vi "axis_angle_to_rotation.vi"(8 "Angle":dbl format="%.5f", 11 "Axis":dbl[](array[numeric])) -> (2 "Rotation":T1=[[1.0, 0.0, 0.0], [0.0, 1.0, 0.0], [0.0, 0.0, 1.0]] format="%#_4g")   [LabVIEW 2013]
uses:
  <vilib>/Analysis/Matrix/Datatypes/RealMatrix.ctl
  norm_vec.vi
  <vilib>/Analysis/Matrix/NI_Matrix.lvlib
panel:
  in  "Zero threshold":dbl=1e-06 format="%.5e"
  # "If angle is less than this, then just return identity, ignoring axis."
  # "Given a unit axis vector and a rotation angle, return the rotation matrix for this 3D rotation."
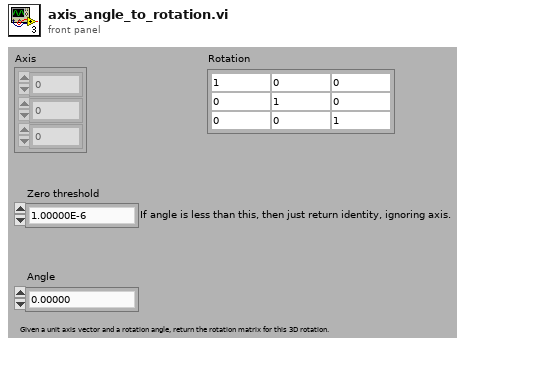
[diagram p1: front panel]
types:
  T1 = typedef "NI_Matrix.lvlib/RealMatrix.ctl" = dbl[][]
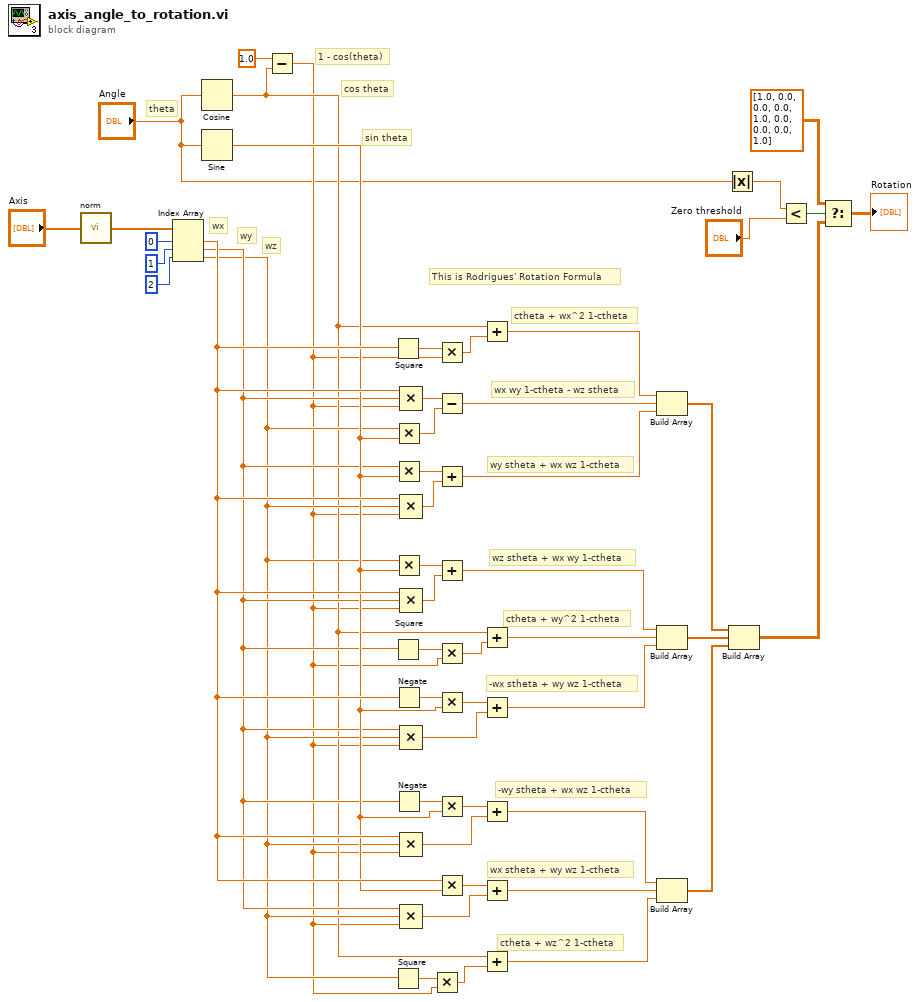
[diagram p0: block diagram]
diagram:
  # "ctheta + wz^2 1-ctheta"
  # "wx stheta + wy wz 1-ctheta"
  # "-wy stheta + wx wz 1-ctheta"
  # "-wx stheta + wy wz 1-ctheta"
  # "ctheta + wy^2 1-ctheta"
  # "wz stheta + wx wy 1-ctheta"
  # "wy stheta + wx wz 1-ctheta"
  # "wx wy 1-ctheta - wz stheta"
  # "ctheta + wx^2 1-ctheta"
  # "sin theta"
  # "cos theta"
  # "wz"
  # "wy"
  # "wx"
  # "1 - cos(theta)"
  # "theta"
  # "This is Rodrigues' Rotation Formula"
  n1 = call-poly "norm.vi"("vector"="Axis") -> ("normalized vector"=w1:dbl[])  [unwired: 3 in, 1 out]
  n2 = Index Array(array=w1, index #1=0 ("index"), index #2=1 ("index"), index #3=2 ("index")) -> (element #1=w24:dbl, element #2=w21:dbl, element #3=w20:dbl)
  n3 = Cosine(x="Angle") -> (cos(x)=w17:dbl)
  n4 = Sine(x="Angle") -> (sin(x)=w23:dbl)
  n5 = Subtract(x=1.0, y=w17) -> (x-y=w15:dbl)
  n6 = Square(x=w24) -> (x^2=w47:dbl)
  n7 = Square(x=w21) -> (x^2=w35:dbl)
  n8 = Square(x=w20) -> (x^2=w16:dbl)
  n9 = Multiply(x=w20, y=w23) -> (x*y=w43:dbl)
  n10 = Multiply(x=w21, y=w23) -> (x*y=w41:dbl)
  n11 = Multiply(x=w20, y=w23) -> (x*y=w38:dbl)
  n12 = Negate(x=w24) -> (-x=w32:dbl)
  n13 = Negate(x=w21) -> (-x=w28:dbl)
  n14 = Compound Arithmetic op=MULTIPLY(w24, w21, w15) -> (w44:dbl)
  n15 = Compound Arithmetic op=MULTIPLY(w24, w20, w15) -> (w40:dbl)
  n16 = Compound Arithmetic op=MULTIPLY(w24, w21, w15) -> (w37:dbl)
  n17 = Compound Arithmetic op=MULTIPLY(w21, w20, w15) -> (w30:dbl)
  n18 = Compound Arithmetic op=MULTIPLY(w24, w20, w15) -> (w26:dbl)
  n19 = Compound Arithmetic op=MULTIPLY(w21, w20, w15) -> (w19:dbl)
  n20 = Multiply(x=w16, y=w15) -> (x*y=w14:dbl)
  n21 = Multiply(x=w47, y=w15) -> (x*y=w46:dbl)
  n22 = Subtract(x=w44, y=w43) -> (x-y=w42:dbl)
  n23 = Add(x=w41, y=w40) -> (x+y=w39:dbl)
  n24 = Add(x=w38, y=w37) -> (x+y=w36:dbl)
  n25 = Multiply(x=w35, y=w15) -> (x*y=w34:dbl)
  n26 = Multiply(x=w32, y=w23) -> (x*y=w31:dbl)
  n27 = Multiply(x=w28, y=w23) -> (x*y=w27:dbl)
  n28 = Multiply(x=w24, y=w23) -> (x*y=w22:dbl)
  n29 = Add(x=w17, y=w46) -> (x+y=w45:dbl)
  n30 = Add(x=w17, y=w34) -> (x+y=w33:dbl)
  n31 = Add(x=w31, y=w30) -> (x+y=w29:dbl)
  n32 = Add(x=w27, y=w26) -> (x+y=w25:dbl)
  n33 = Add(x=w22, y=w19) -> (x+y=w18:dbl)
  n34 = Add(x=w17, y=w14) -> (x+y=w13:dbl)
  n35 = Build Array(w45, w42, w39) -> (w12:dbl[])
  n36 = Build Array(w36, w33, w29) -> (w11:dbl[])
  n37 = Build Array(w25, w18, w13) -> (w10:dbl[])
  n38 = Absolute Value(x="Angle") -> (abs(x)=w8:dbl)
  n39 = Build Array(w12, w11, w10) -> (w4:dbl[][])
  n40 = Less?(x=w8, y="Zero threshold") -> (x < y?=w6:bool)
  n41 = Select(t=dbl[][] [[1.0, 0.0, 0.0], [0.0, 1.0, 0.0], [0.0, 0.0, 1.0]] ("appended array"), s=w6, f=w4) -> (s? t:f=→"Rotation":dbl[][])
